vi "Launch jettl Queue Actor.vi"(9 "Alias":string, 10 "Queue Actor":refnum<class "Queue Actor.lvclass">) -> ()   [LabVIEW 2021, in "jettl.lvlib" / "jettl Queue Actor.lvlib" / "jettl Queue Actor.lvclass"]
uses:
  jettl Queue Actor.lvclass
  jettl Queue Actor.lvclass/jettl Queue Actor.ctl
  jettl.lvlib
  State/Teardown State/Teardown State.lvclass
  Actor/Queue Actor/Queue Actor.lvclass
  C:/git/jettl/src/Actor/Actor/Actor.lvclass
  C:/git/jettl/src/Actor/Msgs/Create/Create/Create.lvclass
  C:/git/jettl/src/Actor/Msgs/Merge Error/Merge Error/Merge Error.lvclass
  C:/git/jettl/src/Actor/Msgs/Override Error/Override Error/Override Error.lvclass
  C:/git/jettl/src/Actor/Msgs/Teardown/Teardown/Teardown.lvclass
  C:/git/jettl/src/Actor/Queue Actor/Queue Actor.lvclass
  C:/git/jettl/src/Actor/Msgs/Last Ack/Last Ack/Last Ack.lvclass
  C:/git/jettl/src/jettl/jettl Queue Actor/jettl Queue Actor/jettl Queue Actor.lvclass
  C:/git/jettl/src/jettl/jettl Queue Actor/State/Teardown State/Teardown State.lvclass
  C:/git/jettl/src/jettl/jettl Queue Actor/State/State/State.lvclass
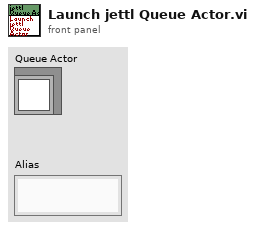
[diagram p1: front panel]
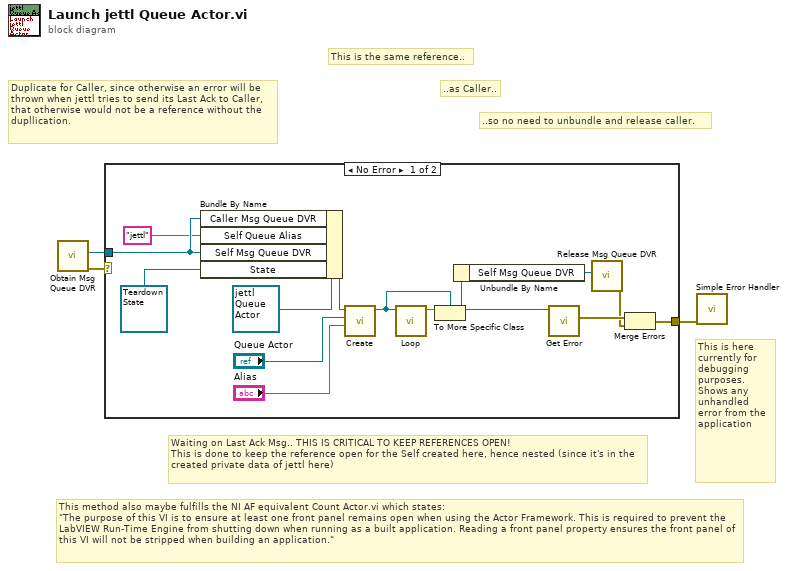
[diagram p0: block diagram]
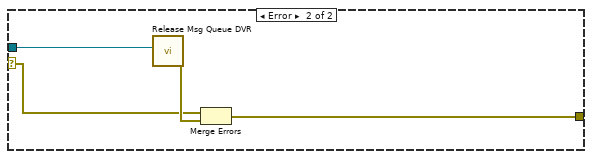
[diagram p2: hidden frame]
diagram:
  # "Duplicate for Caller, since otherwise an error will be thrown when jettl tries to send its Last Ack to Caller, that otherwise would not be a reference without the dupllication."
  # "..so no need to unbundle and release caller."
  # "This is the same reference.."
  # "..as Caller.."
  # "Waiting on Last Ack Msg.. THIS IS CRITICAL TO KEEP REFERENCES OPEN!\nThis is done to keep the reference open for the Self created here, hence nested (since it's in the created private data of jettl here)"
  # "This method also maybe fulfills the NI AF equivalent Count Actor.vi which states:\n\"The purpose of this VI is to ensure at least one front panel remains open when using the Actor Framework. This is required to prevent the LabVIEW Run-Time Engine from shutting down when running as a built application. Reading a front panel property ensures the front panel of this VI will not be stripped when building an application.\""
  # "This is here currently for debugging purposes.\nShows any unhandled error from the application"
  n1 = call "Obtain Msg Queue DVR.vi"() -> ("error out"=w1:errorcluster, "Msg Queue DVR"=w3:refnum<data-value>)  [unwired: 10 in]
  n2 = case shown="No Error" w1 {
    selector: w1 -> [_ w18]
    tunnel: w3 -> [w5 w21]
    tunnel: [w16 w20] -> w2
    frame No Error {
      n3 = Bundle By Name(cluster=refnum<class "jettl Queue Actor.lvclass"> refnum ("Self Actor in"), "Caller Msg Queue DVR"=w5, "Self Queue Alias"="jettl" ("Self Alias"), "Self Msg Queue DVR"=w5, "State"=refnum<class "Teardown State.lvclass"> refnum ("jettl.lvlib:Destroy State.lvclass")) -> (w15:refnum<class "jettl Queue Actor.lvclass">)
      n4 = call-dynamic "Create.vi"("Alias"="Alias", "Actor"="Queue Actor", "jettl Queue Actor in"=w15) -> ("jettl Queue Actor out"=w7:refnum<class "jettl Queue Actor.lvclass">)  [unwired: 8 in]
      n5 = call "Loop.vi"(11:w7) -> (3:w8)  [unwired: 10 in]
      n6 = To More Specific Class(target class=w7, reference=w8) -> (specific class reference=w9:refnum<class "jettl Queue Actor.lvclass">)  [unwired: 1 in, 1 out]
      n7 = Unbundle By Name(w9) -> ("Self Msg Queue DVR"=w17:refnum<data-value>)
      n8 = call-dynamic "Get Error.vi"("jettl Queue Actor in"=w9) -> ("Error"=w11:errorcluster)  [unwired: 10 in]
      n9 = call "Release Msg Queue DVR.vi"("Msg Queue DVR"=w17) -> ("error out"=w10:errorcluster)  [unwired: 10 in]
      n10 = Merge Errors(w11, w10) -> (w16:errorcluster)
    }
    frame Error {
      n11 = call "Release Msg Queue DVR.vi"("Msg Queue DVR"=w21) -> ("error out"=w19:errorcluster)  [unwired: 10 in]
      n12 = Merge Errors(w18, w19) -> (w20:errorcluster)
    }
  }
  n13 = call <vilib>:"Simple Error Handler.vi"("error in (no error)"=w2) -> ()  [unwired: 4 in, 5 out]
